vi "Call Function with No Arguments.vi"(8 "error in (no error)":errorcluster) -> (0 "error out":errorcluster)   [LabVIEW 2020]
uses:
  908d8fb0-7b42-46e8-9e96-a0c6d44c2c93.vi
  G-Embedded-Python-Interpreter-Toolkit/Null Py Object Refnum.vi
  908d8fb0-7b42-46e8-9e96-a0c6d44c2c93.vi/96ddca92-7bbf-40e2-a1a5-d32f291eb6af.vi
  G-Embedded-Python-Interpreter-Toolkit/Pointer Sized Ref to Python Object Reference.vi
  G-Embedded-Python-Interpreter-Toolkit/Generate Function Call Argument Info.vi
  G-Embedded-Python-Interpreter-Toolkit/Bad Type Error.vi
  G-Embedded-Python-Interpreter-Toolkit/Generate Function Call Argument Info.vi/5ba79b4d-2978-48e4-80f3-d9d30d92ebfd.vi
  G-Embedded-Python-Interpreter-Toolkit/Merge Call Library Errors.vi
  <vilib>/Utility/Data Type/Get Type Information.vi
  <vilib>/Utility/error.llb/Error Cluster From Error Code.vi
  <vilib>/Utility/Data Type/Get Cluster Information.vi
  <vilib>/Utility/Data Type/Get Array Information.vi
  <vilib>/addons/_JKI Toolkits/Caraya/classes/Assert/Assert Not Error.vi
  <vilib>/addons/_JKI Toolkits/Caraya/classes/Assert/Assert Equal Value and Type_Variant.vi
  <vilib>/Comparison/Equal/Equal Functor/Equal Functor.lvclass
  G-Embedded-Python-Interpreter-Toolkit/G-Embedded-Python-Interpreter-Toolkit.lvlib
  <vilib>/addons/_JKI Toolkits/Caraya/classes/Test/Test.lvclass
  <vilib>/addons/_JKI Toolkits/Caraya/classes/Assert/Assert.lvclass
panel:
  out "Value":i32
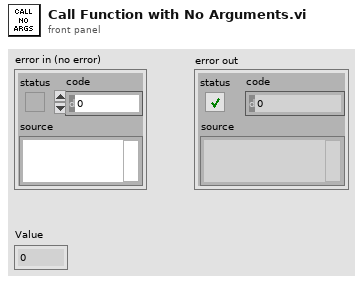
[diagram p1: front panel]
types:
  T1 = typedef "G-Embedded-Python-Interpreter-Toolkit.lvlib/Python Object Reference.ctl" = refnum<k1>
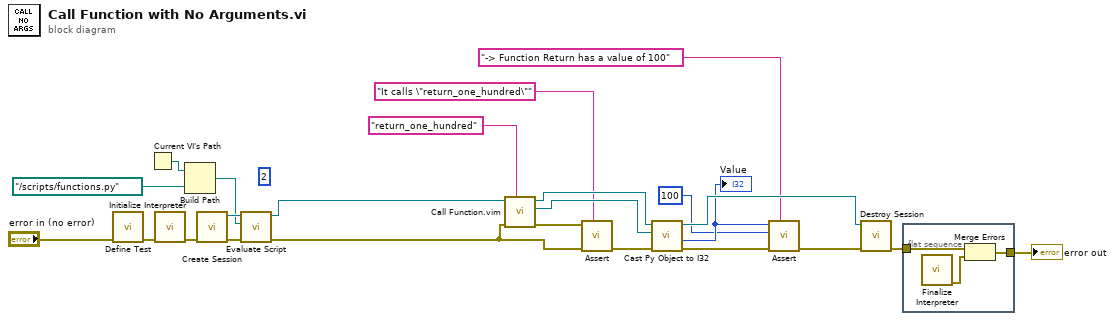
[diagram p0: block diagram]
diagram:
  (unwired) 2
  n1 = call <vilib>:"Define Test.vi"("error in (no error)"="error in (no error)") -> ("error out"=w24:errorcluster)  [unwired: 10 in]
  n2 = Current VI's Path() -> (path=w19:path)
  n3 = call "Initialize Interpreter.vi"("error in (no error)"=w24) -> ("error out"=w21:errorcluster)  [unwired: 9 in, 1 out]
  n4 = Build Path(base path=w19, name or relative path=path "../scripts/functions.py" ("Path")) -> (appended path=w17:path)
  n5 = call "Create Session.vi"("error in (no error)"=w21) -> ("error out"=w16:errorcluster, "Session Handle"=w20:refnum<data-value>)  [unwired: 9 in]
  n6 = call "Evaluate Script.vi"("error in (no error)"=w16, "Script File Path"=w17, "Session Handle in"=w20) -> ("error out"=w2:errorcluster, "Session Handle out"=w1:refnum<data-value>)  [unwired: 7 in]
  n7 = call "Call Function.vim"("Function Name"="return_one_hundred", "error in (no error)"=w2, "Data Value Reference in"=w1) -> ("error out"=w6:errorcluster, "Returned Python Object Refnum"=w13:T1, "Data Value Reference out"=w14:refnum<data-value>)  [unwired: 6 in]
  n8 = call-poly <vilib>:"Assert.vi"("Label"="It calls \"return_one_hundred\"", "error in (no error)"=w2, "Not Error?"=w6) -> ("error out"=w5:errorcluster)  [unwired: 8 in]
  n9 = call "Cast Py Object to I32.vi"("error in (no error)"=w5, "Python Object Refnum in"=w13, "Session Handle in"=w14) -> ("error out"=w4:errorcluster, "Value"=w11:i32, "Session Handle out"=w12:refnum<data-value>)  [unwired: 5 in, 1 out]
  "Value" <- w11
  n10 = call-poly <vilib>:"Assert.vi"("Label"="-> Function Return has a value of 100", "error in (no error)"=w4, "Y"=100 ("Value"), "X"=w11) -> ("error out"=w10:errorcluster)  [unwired: 7 in]
  n11 = call "Destroy Session.vi"("error in (no error)"=w10, "Session Handle"=w12) -> ("error out"=w15:errorcluster)  [unwired: 9 in]
  n12 = flat-sequence {
    tunnel: w15 -> [w27]
    tunnel: [w25] -> w22
    frame #0 {
      n13 = call "Finalize Interpreter.vi"() -> ("error out"=w26:errorcluster)  [unwired: 11 in]
      n14 = Merge Errors(w27, w26) -> (w25:errorcluster)
    }
  }
  "error out" <- w22
